vi "daq_FSM.vi"(8 "error in (no error)":errorcluster, 10 "Measures":refnum<queue>, 11 "Commands":refnum<queue>) -> ()   [LabVIEW 2019]
uses:
  <vilib>/DAQmx/read.llb/DAQmx Read (Analog 1D DBL 1Chan NSamp).vi
  <vilib>/DAQmx/miscellaneous.llb/DAQmx Fill In Error Info.vi
panel:
  in  "Configuration":T1={"Sampling"={"Samples per channel"=0, "Sample rate"=0.0}, "Acquisition"={"physical channels"="", "sample mode"=10178, "Min Val."=0.0, "Max Val."=0.0}} {"Acquisition"."sample mode" items=["Finite Samples"=10178, "Continuous Samples"=10123, "Hardware Timed Single Point"=12522]}
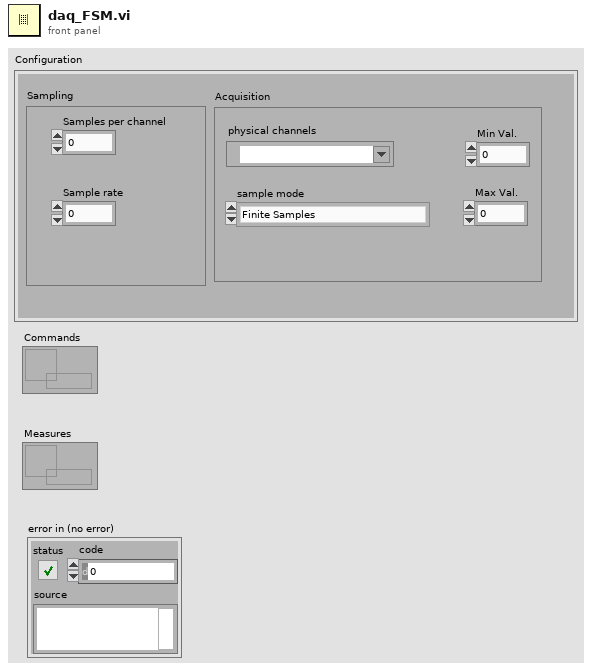
[diagram p1: front panel]
types:
  T1 = cluster{"Sampling":cluster{"Samples per channel":i32, "Sample rate":dbl}, "Acquisition":cluster{"physical channels":tag, "sample mode":i32, "Min Val.":dbl, "Max Val.":dbl}}
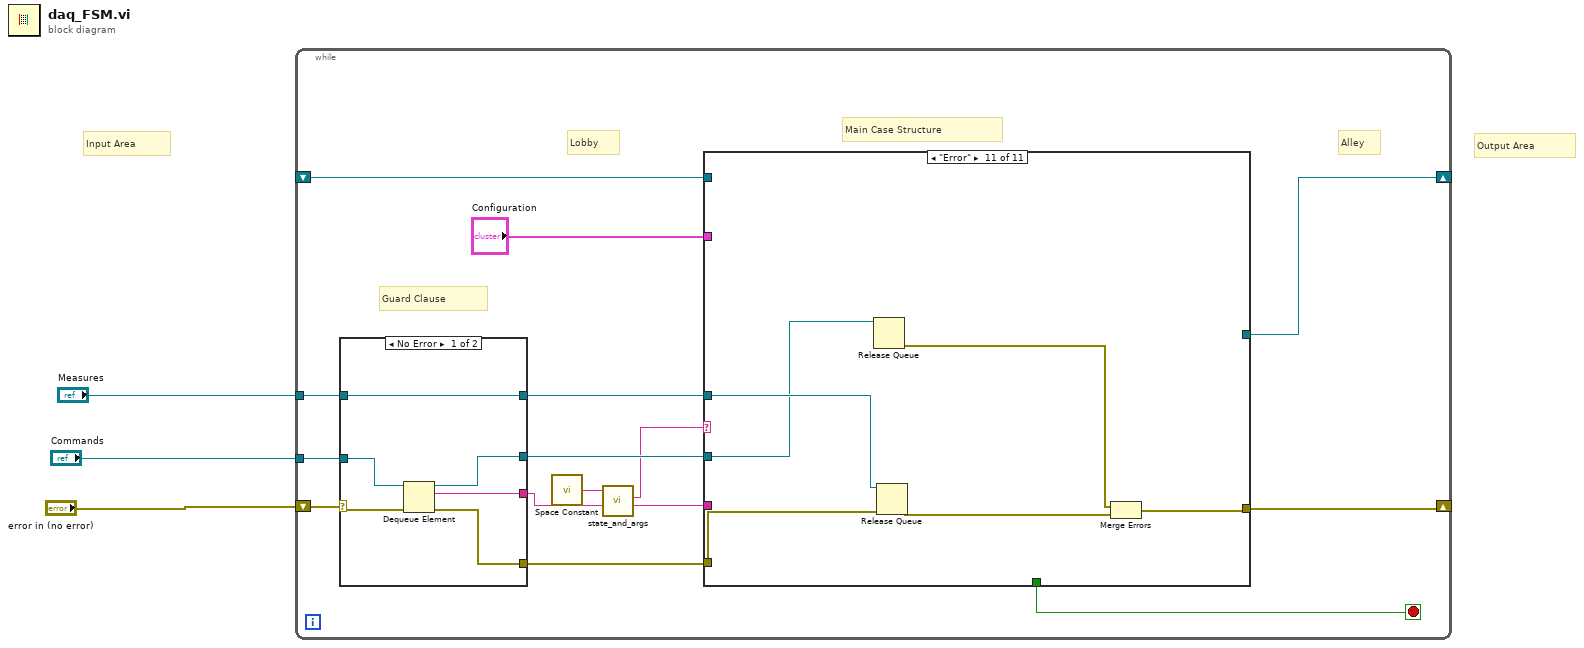
[diagram p0: block diagram]
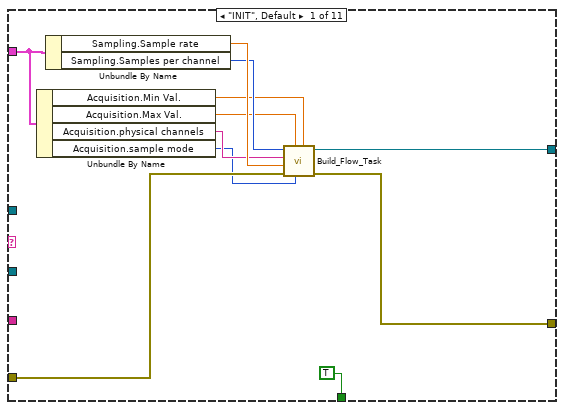
[diagram p2: hidden frame]
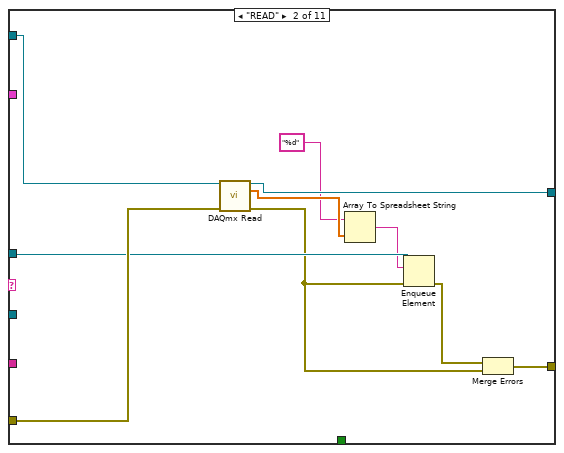
[diagram p3: hidden frame]
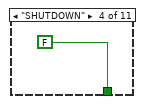
[diagram p5: hidden frame]
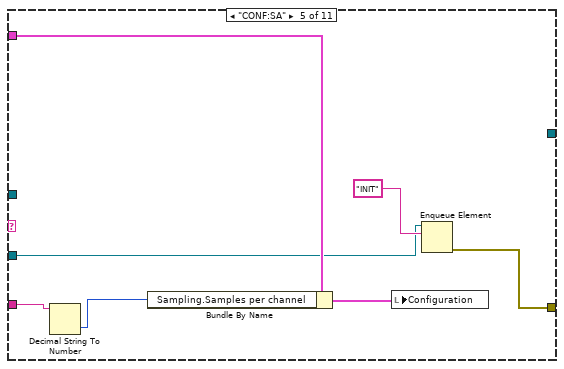
[diagram p6: hidden frame]
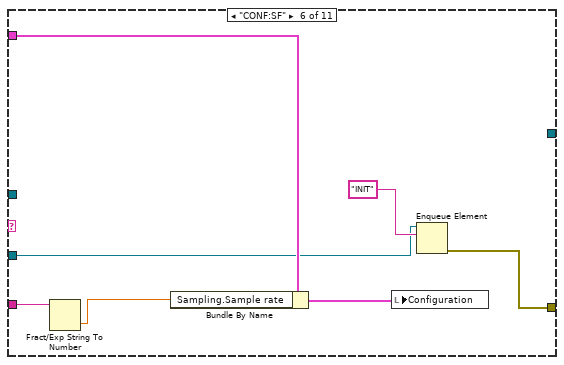
[diagram p7: hidden frame]
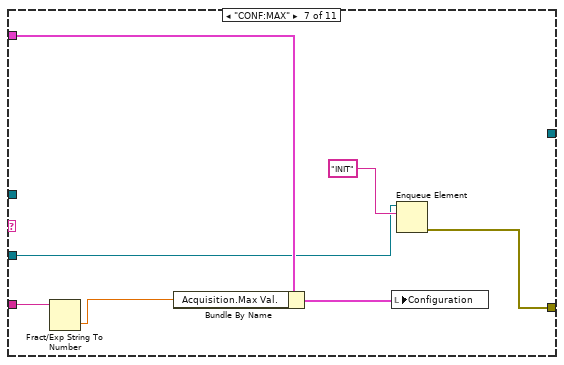
[diagram p8: hidden frame]
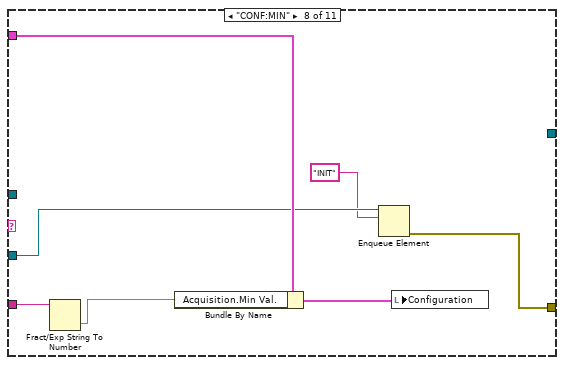
[diagram p9: hidden frame]
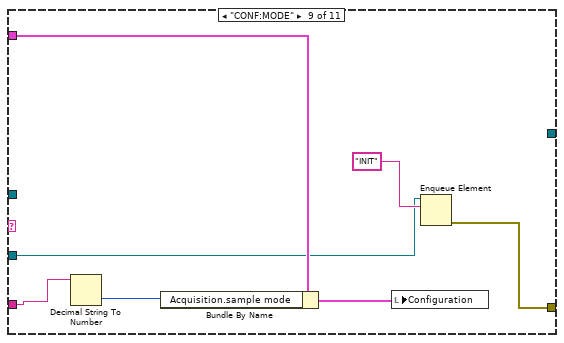
[diagram p10: hidden frame]
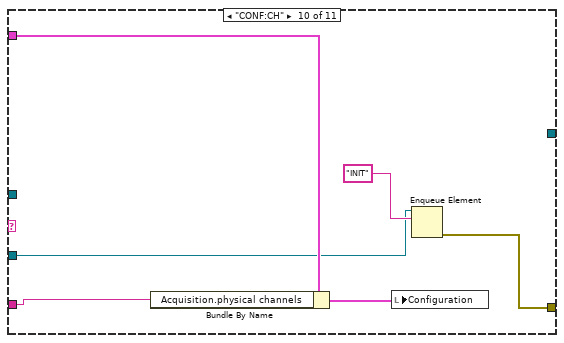
[diagram p11: hidden frame]
diagram:
  # "Output Area"
  # "Input Area"
  n1 = while {
    shift-right: [w12] -> _
    shift-left: "error in (no error)" -> [w18]
    tunnel: "Commands" -> [w17]
    tunnel: "Measures" -> [w16]
    shift-right: [w9] -> _
    shift-left: _ -> [w8]
    stop <- w10 stop-if-true
    # "Lobby"
    # "Alley"
    # "Main Case Structure"
    # "Guard Clause"
    n2 = case shown="No Error" w18 {
      selector: w18 -> [w94 w95]
      tunnel: w17 -> [w93 _]
      tunnel: [w92 _] -> w7
      tunnel: [w91 _] -> w14
      tunnel: [w90 w95] -> w13
      tunnel: [w89 _] -> w15
      tunnel: w16 -> [w89 _]
      frame No Error {
        n3 = Dequeue Element(queue=w93, error in (no error)=w94) -> (queue out=w91:refnum<queue>, element=w92:string, error out=w90:errorcluster)  [unwired: 1 in, 1 out]
      }
      frame Error {
      }
    }
    n4 = call <vilib>:"Space Constant.vi"() -> ("String"=w6:string)
    n5 = call "state_and_args.vi"("String"=w7, "DELIMITER (:)"=w6) -> ("Arguments"=w4:string, "State"=w5:string)  [unwired: 8 in]
    n6 = case shown="\"Error\"" w5 {
      tunnel: w15 -> [_ w36 _ _ _ _ _ _ _ _ w87]
      tunnel: w14 -> [_ _ _ _ w43 w50 w57 w65 w71 w78 w83]
      tunnel: w13 -> [w29 w37 w40 _ _ _ _ _ _ _ w88]
      tunnel: [w28 w31 w40 _ w42 w49 w56 w63 w70 w77 w86] -> w12
      tunnel: "Configuration" -> [w25 _ _ _ w48 w55 w62 w69 w76 w82 _]
      tunnel: [TRUE _ _ FALSE _ _ _ _ _ _ _] -> w10
      tunnel: [w19 w38 _ _ _ _ _ _ _ _ _] -> w9
      tunnel: w8 -> [_ w39 _ _ _ _ _ _ _ _ _]
      tunnel: w4 -> [_ _ _ _ w46 w53 w60 w67 w73 w80 _]
      frame "INIT", Default {
        n7 = Unbundle By Name(w25) -> ("Acquisition.Min Val."=w21:dbl, "Acquisition.Max Val."=w22:dbl, "Acquisition.physical channels"=w24:tag, "Acquisition.sample mode"=w23:i32)
        n8 = Unbundle By Name(w25) -> ("Sampling.Sample rate"=w27:dbl, "Sampling.Samples per channel"=w26:i32)
        n9 = call "Build_Flow_Task.vi"("minimum value"=w21, "sample mode"=w23, "maximum value"=w22, "error in"=w29, "rate"=w27, "physical channels"=w24, "samples per channel"=w26) -> ("error out"=w28:errorcluster, "task out"=w19:refnum<k21>)  [unwired: 3 in]
      }
      frame "READ" {
        n10 = call-poly <vilib>:"DAQmx Read.vi"("task/channels in"=w39, "error in"=w37) -> ("task out"=w38:refnum<k21>, "data"=w35:dbl[], "error out"=w30:errorcluster)  [unwired: 11 in]
        n11 = Array To Spreadsheet String(array=w35, 3:"%d" ("format string")) -> (spreadsheet string=w34:string)  [unwired: 1 in]
        n12 = Enqueue Element(queue=w36, element=w34, error in (no error)=w30) -> (error out=w32:errorcluster)  [unwired: 1 in, 2 out]
        n13 = Merge Errors(w32, w30) -> (w31:errorcluster)
      }
      frame "STOP" {
      }
      frame "SHUTDOWN" {
      }
      frame "CONF:SA" {
        n14 = Decimal String To Number(string=w46) -> (number=w45:i32)  [unwired: 2 in, 1 out]
        n15 = Bundle By Name(cluster=w48, "Sampling.Samples per channel"=w45) -> (w47:T1)
        n16 = local write "Configuration"(w47) -> ()
        n17 = Enqueue Element(queue=w43, element="INIT") -> (error out=w42:errorcluster)  [unwired: 2 in, 2 out]
      }
      frame "CONF:SF" {
        n18 = Fract/Exp String To Number(string=w53) -> (number=w52:dbl)  [unwired: 3 in, 1 out]
        n19 = Bundle By Name(cluster=w55, "Sampling.Sample rate"=w52) -> (w54:T1)
        n20 = local write "Configuration"(w54) -> ()
        n21 = Enqueue Element(queue=w50, element="INIT") -> (error out=w49:errorcluster)  [unwired: 2 in, 2 out]
      }
      frame "CONF:MAX" {
        n22 = Fract/Exp String To Number(string=w60) -> (number=w59:dbl)  [unwired: 3 in, 1 out]
        n23 = Bundle By Name(cluster=w62, "Acquisition.Max Val."=w59) -> (w61:T1)
        n24 = local write "Configuration"(w61) -> ()
        n25 = Enqueue Element(queue=w57, element="INIT") -> (error out=w56:errorcluster)  [unwired: 2 in, 2 out]
      }
      frame "CONF:MIN" {
        n26 = Fract/Exp String To Number(string=w67) -> (number=w66:dbl)  [unwired: 3 in, 1 out]
        n27 = Bundle By Name(cluster=w69, "Acquisition.Min Val."=w66) -> (w68:T1)
        n28 = Enqueue Element(queue=w65, element="INIT") -> (error out=w63:errorcluster)  [unwired: 2 in, 2 out]
        n29 = local write "Configuration"(w68) -> ()
      }
      frame "CONF:MODE" {
        n30 = Decimal String To Number(string=w73) -> (number=w74:i32)  [unwired: 2 in, 1 out]
        n31 = Bundle By Name(cluster=w76, "Acquisition.sample mode"=w74) -> (w75:T1)
        n32 = local write "Configuration"(w75) -> ()
        n33 = Enqueue Element(queue=w71, element="INIT") -> (error out=w70:errorcluster)  [unwired: 2 in, 2 out]
      }
      frame "CONF:CH" {
        n34 = Bundle By Name(cluster=w82, "Acquisition.physical channels"=w80) -> (w81:T1)
        n35 = local write "Configuration"(w81) -> ()
        n36 = Enqueue Element(queue=w78, element="INIT") -> (error out=w77:errorcluster)  [unwired: 2 in, 2 out]
      }
      frame "Error" {
        n37 = Release Queue(queue=w83) -> (error out=w84:errorcluster)  [unwired: 2 in, 2 out]
        n38 = Release Queue(queue=w87, error in (no error)=w88) -> (error out=w85:errorcluster)  [unwired: 1 in, 2 out]
        n39 = Merge Errors(w84, w85) -> (w86:errorcluster)
      }
    }
  }
